vi "Dashboard Main.vi"() -> ()   [LabVIEW 2011]
uses:
  2898 Robot Code/TypeDefs/Dashboard Data TypeDef.ctl
  <vilib>/Rock Robotics/WPI/Camera/WPI_CameraImageSize.ctl
panel:
  out "Mode":enum8{"Tele-Op", "Auto", ""}(ring)=enum."Auto"
  in  "Hybrid Close":T1={"Left"=138, "Top"=0, "Right"=209, "Bottom"=45}
  out "Kinect Angle":dbl
  out "FIRE!!!!!":bool
  out "Arms in Correct Position?":bool
  out "Right Y":dbl(slide) scale=-1.0..1.0
  out "Distance Away from Player (Feet)":dbl
  out "Left Y":dbl(slide) scale=-1.0..1.0
  out "Is Kinect Override Enabled?":bool
  out "Is Kinect Enabled?":bool
  in  "Teleop":T1={"Left"=144, "Top"=36, "Right"=201, "Bottom"=76}
  in  "stop":bool
  out "Aligning Mode?":bool
  out "Bridge Mode?":bool
  in  "Ball Count Down":bool
  in  "Ball Count Up":bool
  out "Number of Balls":i32=2
  out "Shooting Manual Override?":bool
  in  "Autonomous Delay":dbl
  in  "Autonomcous Mode":T2(ring) caption="Autonomous Mode"
  out "Ball Collection":bool
  out "Shooter":bool=TRUE
  out "Shooter At Speed?":bool
  out "Ball Camera":T3(plugin-control)
  out "Image Error Message 2":string="Timeout in Camera Communications"
  out "Target Camera":T3(plugin-control)
  out "Dashboard Datatype Warning":string="Warning: The Dashboard Datatype used by the robot project and this dashboard do not match.\nSee diagram for more details."
  out "Robot IP Address":string="10.15.10.2"
  out "Image Error Message":string="Timeout in Camera Communications"
  # "Communications"
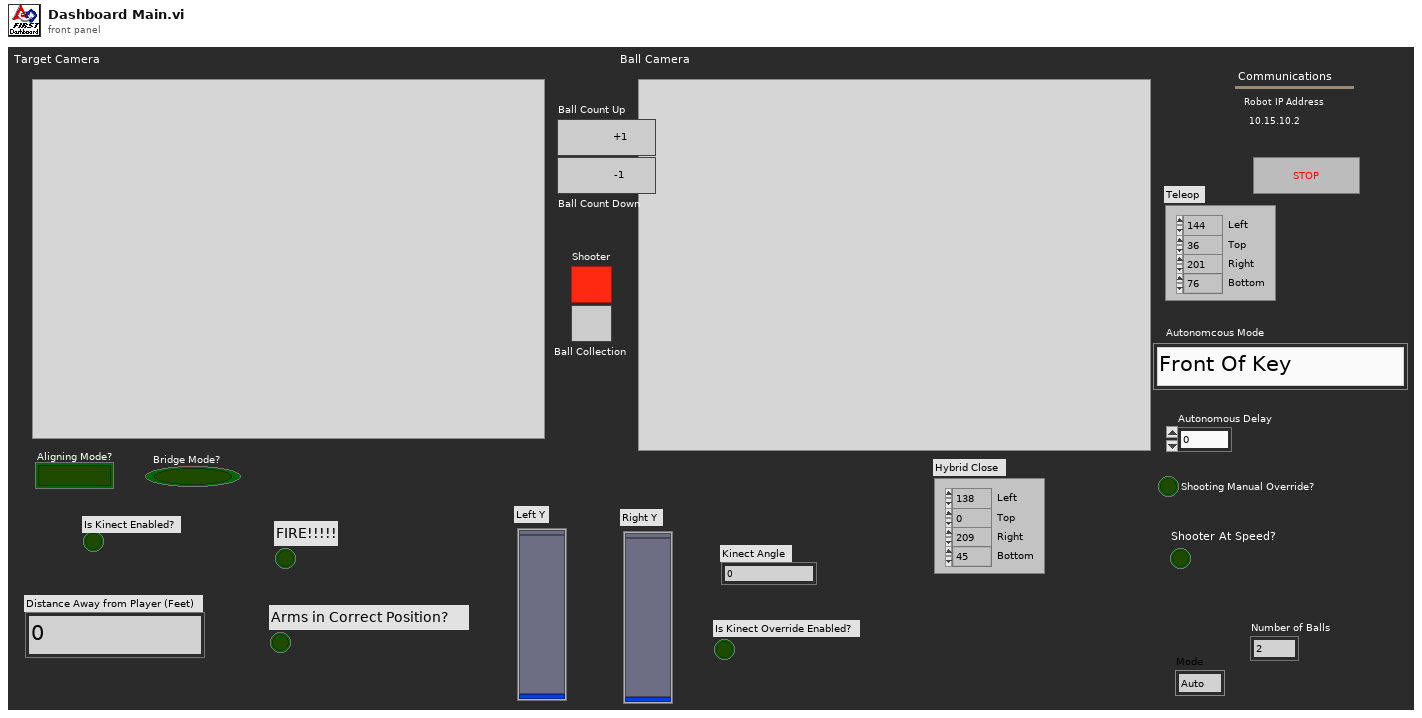
[diagram p1: front panel]
types:
  T1 = cluster{"Left":i32, "Top":i32, "Right":i32, "Bottom":i32}
  T2 = enum16{"Front Of Key", "Middle of Key (SEA)", "Back of Key", "Bridge", "Disable"}
  T3 = typedef "IMAQ Image.ctl" = refnum<image>
  T4 = typedef "Image Type" = u32
  T5 = cluster{"Ball Count Up":bool, "Ball Count Down":bool}
  T6 = cluster{"Autonomous Delay":dbl, "Autonomcous Mode":enum16{"Front Of Key", "Middle of Key (SEA)", "Back of Key", "Bridge", "Disable"}}
  T7 = cluster{cluster{"Ball Count Up":bool, "Ball Count Down":bool}, cluster{"Autonomous Delay":dbl, "Autonomcous Mode":enum16{"Front Of Key", "Middle of Key (SEA)", "Back of Key", "Bridge", "Disable"}}}
  T8 = typedef "Vector4.ctl" = cluster{"x":sgl, "y":sgl, "z":sgl, "w":sgl}
  T9 = typedef "SkeletonTrackState.ctl" = enum32{"NotTracked", "PositionOnly", "Tracked"}
  T10 = typedef "WPI_JoystickDeviceDataRaw.ctl" = cluster{"axis 1":i8, "axis 2":i8, "axis 3":i8, "axis 4":i8, "axis 5":i8, "axis 6":i8, "Buttons":u16}
  T11 = cluster{cluster{"Version String":string, "Number of Players":i8, "Flags":u32, "FloorClipPlane":T8, "Gravity Normal":cluster{"x":sgl, "y":sgl, "z":sgl}}, cluster{"TrackingState":u8[], "Overall Position":cluster{"x":sgl, "y":sgl, "z":sgl}, "Quality":u32, "TrackState":T9}, "Skeleton Vertices":cluster{"x":sgl, "y":sgl, "z":sgl}[], "Joystick":T10, "Joystick 2":T10, "Custom Data":string}
  T12 = typedef "Dashboard Data TypeDef.ctl" = cluster{"Number of Balls":i32, "Shooting Manual Override?":bool, "Bridge Mode?":bool, "Shooter":bool, "Shooter At Speed?":bool, "Aligning Mode?":bool}
  T13 = cluster{"Competition mode":bool, "Robot Link":bool, "Autonomous":bool, "Enabled":bool, "E-Stop":bool}
  T14 = typedef "WPI_CameraImageSize.ctl" = enum16{"640x480", "320x240", "160x120"}
  T15 = cluster{"fps":i32, "compression":i32, "Image Size":T14}
  T16 = typedef "LVRectTypeDef.ctl" = cluster{"left":i16, "top":i16, "right":i16, "bottom":i16}
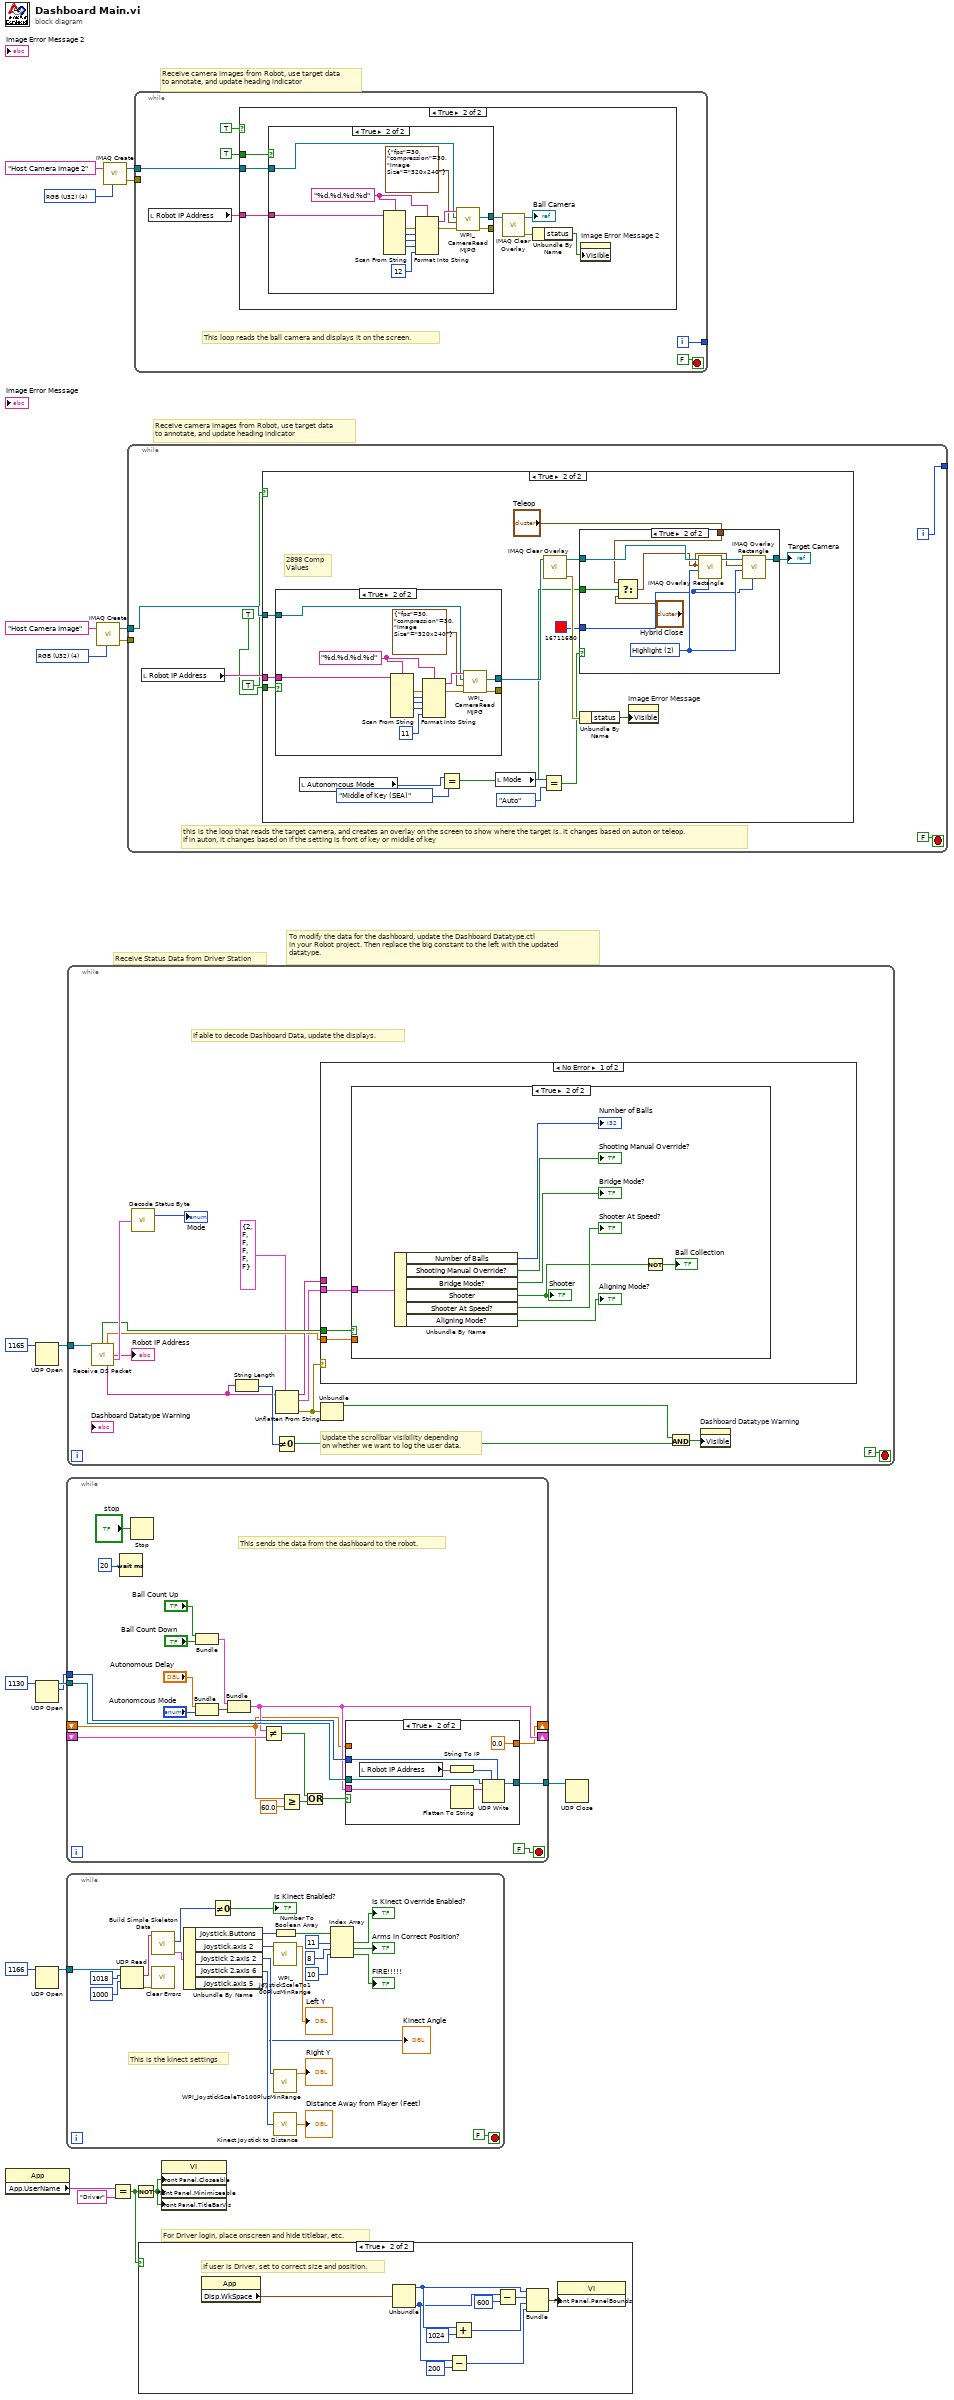
[diagram p0: block diagram]
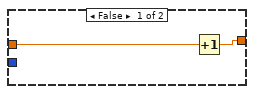
[diagram p2: hidden frame]
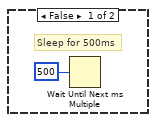
[diagram p3: hidden frame]
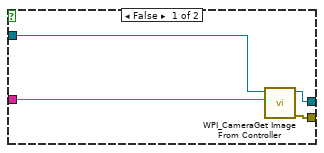
[diagram p4: hidden frame]
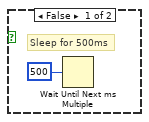
[diagram p8: hidden frame]
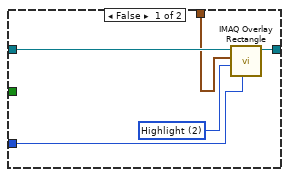
[diagram p9: hidden frame]
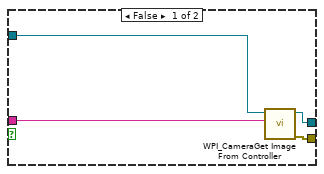
[diagram p10: hidden frame]
diagram:
  w8 = T4 4 items=["Grayscale (U8)", "Grayscale (I16)", "Grayscale (SGL)", "Complex (CSG)", "RGB (U32)", "HSL (U32)", "RGB (U64)"] ("Image Type")
  w18 = T4 4 items=["Grayscale (U8)", "Grayscale (I16)", "Grayscale (SGL)", "Complex (CSG)", "RGB (U32)", "HSL (U32)", "RGB (U64)"] ("Image Type")
  # "Receive camera images from Robot, use target data\nto annotate, and update heading indicator"
  # "For Driver login, place onscreen and hide titlebar, etc."
  # "To modify the data for the dashboard, update the Dashboard Datatype.ctl\nin your Robot project. Then replace the big constant to the left with the updated\ndatatype."
  # "Receive Status Data from Driver Station"
  # "Receive camera images from Robot, use target data\nto annotate, and update heading indicator"
  n1 = property class="App"() -> ("App.UserName"=w13:string)  [unwired: 2 in, 2 out]
  n2 = UDP Open(11:u16 1165 ("port")) -> (port=w19:refnum<k16>)  [unwired: 2 in, 4 out]
  n3 = UDP Open(11:u16 1130 ("port")) -> (port=w7:refnum<k16>, 2:w6:u16)  [unwired: 4 in, 1 out]
  n4 = UDP Open(11:u16 1166 ("port")) -> (port=w1:refnum<k16>)  [unwired: 2 in, 4 out]
  n5 = while {
    tunnel: w7 -> [w36]
    tunnel: w6 -> [w35]
    tunnel: [w34] -> w5
    shift-right: [w33] -> _
    shift-left: _ -> [w32]
    shift-right: [w29] -> _
    shift-left: _ -> [w26]
    stop <- FALSE stop-if-true
    # "This sends the data from the dashboard to the robot."
    n6 = Wait (ms)(milliseconds to wait=u32 20) -> ()  [unwired: 1 out]
    n7 = Stop(stop? (T)="stop") -> ()
    n8 = Bundle("Ball Count Up"="Ball Count Up", "Ball Count Down"="Ball Count Down") -> (w38:T5)  [unwired: 1 in]
    n9 = Bundle("Autonomous Delay"="Autonomous Delay", "Autonomcous Mode"="Autonomcous Mode") -> (w37:T6)  [unwired: 1 in]
    n10 = Bundle(w38, w37) -> (w33:T7)  [unwired: 1 in]
    n11 = Not Equal?(x=w33, y=w32) -> (x != y?=w25:bool)
    n12 = Greater Or Equal?(x=w26, y=60.0) -> (x >= y?=w27:bool)
    n13 = Or(x=w25, y=w27) -> (x .or. y?=w24:bool)
    n14 = case shown="True" w24 {
      tunnel: w33 -> [_ w50]
      tunnel: w36 -> [_ w48]
      tunnel: w35 -> [_ w47]
      tunnel: [_ w46] -> w34
      tunnel: [w42 0.0] -> w29
      tunnel: w26 -> [w41 _]
      frame False {
        n15 = Increment(x=w41) -> (x+1=w42:dbl)
      }
      frame True {
        n16 = local read "Robot IP Address"() -> (w44:string)
        n17 = String To IP(1:w44) -> (0:w45:u32)
        n18 = Flatten To String(anything=w50) -> (data string=w49:string)  [unwired: 3 in, 2 out]
        n19 = UDP Write(address=w45, port or service name=w47, connection ID=w48, data in=w49) -> (3:w46:refnum<k16>)  [unwired: 2 in, 1 out]
      }
    }
  }
  n20 = while {
    tunnel: w1 -> [w72]
    stop <- FALSE stop-if-true
    # "This is the kinect settings"
    n21 = UDP Read(connection ID=w72, max size (548)=1018 ("bytes to read"), timeout ms (25000)=1000) -> (data out=w71:string, error out=w62:errorcluster)  [unwired: 1 in, 3 out]
    n22 = call "Build Simple Skeleton Data.vi"("data out"=w71) -> ("Kinect Outputs"=w68:T11, "NumPlayers"=w70:i8)  [unwired: 6 in, 3 out]
    n23 = call <vilib>:"Clear Errors.vi"("error in (no error)"=w62) -> ()  [unwired: 6 in, 1 out]
    n24 = Unbundle By Name(w68) -> ("Joystick.Buttons"=w67:u16, "Joystick.axis 2"=w59:i8, "Joystick 2.axis 2"=w58:i8, "Joystick 2.axis 6"=w61:i8, "Joystick.axis 5"=→"Kinect Angle":i8)
    n25 = Not Equal To 0?(x=w70) -> (x != 0?=→"Is Kinect Enabled?":bool)
    n26 = call <vilib>:"WPI_JoystickScaleTo100PlusMinRange.vi"("RawValue"=w59) -> ("ScaledToPercentRange"=→"Left Y":dbl)  [unwired: 1 in, 9 out]
    n27 = call <vilib>:"WPI_JoystickScaleTo100PlusMinRange.vi"("RawValue"=w58) -> ("ScaledToPercentRange"=→"Right Y":dbl)  [unwired: 1 in, 9 out]
    n28 = call "Kinect Joystick to Distance.vi"("Input"=w61) -> ("Output"=→"Distance Away from Player (Feet)":dbl)
    n29 = Number To Boolean Array(number=w67) -> (Boolean array=w66:bool[])
    n30 = Index Array(array=w66, index #1=11 ("index"), index #2=8 ("index"), index #3=10 ("index")) -> (element #1=→"Is Kinect Override Enabled?":bool, element #2=→"Arms in Correct Position?":bool, element #3=→"FIRE!!!!!":bool)
  }
  n31 = while {
    tunnel: w19 -> [w89]
    stop <- FALSE stop-if-true
    # "Update the scrollbar visibility depending\non whether we want to log the user data."
    # "If able to decode Dashboard Data, update the displays."
    n32 = call "Receive DS Packet.vi"("Recv Socket"=w89) -> ("New Dashboard Data"=w87:bool, "Battery"=w80:sgl, "Robot IP Address"=→"Robot IP Address":string, "Status"=w90:T13, "High Priority User Data"=w77:string)  [unwired: 1 in, 9 out]
    n33 = call "Decode Status Byte.vi"("Status Byte"=w90) -> ("Mode"=→"Mode":enum8{"Tele-Op", "Auto", ""})  [unwired: 1 out]
    n34 = String Length(string=w77) -> (length=w82:i32)
    n35 = Not Equal To 0?(x=w82) -> (x != 0?=w85:bool)
    n36 = Unflatten From String(type=T12 {"Number of Balls"=2, "Shooting Manual Override?"=FALSE, "Bridge Mode?"=FALSE, "Shooter"=FALSE, "Shooter At Speed?"=FALSE, "Aligning Mode?"=FALSE} ("Cluster"), binary string=w77) -> (rest of the binary string=w83:string, value=w79:T12, error out=w88:errorcluster)  [unwired: 1 in, 2 out]
    n37 = case shown="No Error" w88 {
      tunnel: w87 -> [w93 _]
      tunnel: w83 -> [_ _]
      tunnel: w80 -> [w92 _]
      tunnel: w79 -> [w91 _]
      frame No Error {
        n38 = case shown="True" w93 {
          tunnel: w92 -> [_ _]
          tunnel: w91 -> [_ w101]
          frame False {
            # "Don't update if the robot hasn't sent new data"
          }
          frame True {
            n39 = Unbundle By Name(w101) -> ("Number of Balls"=→"Number of Balls":i32, "Shooting Manual Override?"=→"Shooting Manual Override?":bool, "Bridge Mode?"=→"Bridge Mode?":bool, "Shooter"=w95:bool, "Shooter At Speed?"=→"Shooter At Speed?":bool, "Aligning Mode?"=→"Aligning Mode?":bool)
            "Shooter" <- w95
            n40 = Not(x=w95) -> (.not. x?=→"Ball Collection":bool)
          }
        }
      }
      frame Error {
        # "Your datatypes don't match. The Dashboard Datatype.ctl in your Robot project\nand the big constant to the left of the loop need to match."
      }
    }
    n41 = Unbundle(w88) -> ("status"=w84:bool)  [unwired: 2 out]
    n42 = And(x=w84, y=w85) -> (x .and. y?=w86:bool)
    n43 = property on="Dashboard Datatype Warning" class="Str"("Visible"=w86) -> ()  [unwired: 2 in, 2 out]
  }
  n44 = call "IMAQ Create"("Image Name"="Host Camera Image", "Image Type"=w18) -> ("New Image"=w16:T3, "error out"=w15:errorcluster)  [unwired: 2 in, 1 out]
  n45 = call "IMAQ Create"("Image Name"="Host Camera Image 2", "Image Type"=w8) -> ("New Image"=w10:T3, "error out"=w11:errorcluster)  [unwired: 2 in, 1 out]
  n46 = Equal?(x=w13, y="Driver") -> (x = y?=w12:bool)
  n47 = while {
    tunnel: w16 -> [w105]
    tunnel: w15 -> [_]
    tunnel: [w103] -> _
    i -> [w103]
    stop <- FALSE stop-if-true
    # "this is the loop that reads the target camera, and creates an overlay on the screen to show where the target is. It changes based on auton or teleop.\nIf in auton, it changes based on if the setting is front of key or middle of key"
    n48 = local read "Robot IP Address"() -> (w106:string)
    n49 = case shown="True" TRUE {
      tunnel: w106 -> [_ w124]
      tunnel: w105 -> [_ w123]
      tunnel: TRUE -> [_ w119]
      frame False {
        # "Sleep for 500ms"
        n50 = Wait Until Next ms Multiple(millisecond multiple=u32 500) -> ()  [unwired: 1 out]
      }
      frame True {
        # "2898 Comp\nValues"
        n51 = case shown="True" w119 {
          tunnel: w123 -> [w141 w149]
          tunnel: [w139 w147] -> _
          tunnel: [w140 w148] -> w120
          tunnel: w124 -> [w142 w152]
          frame False {
            n52 = call <vilib>:"WPI_CameraGet Image From Controller.vi"("Controller Address"=w142, "Image"=w141) -> ("error out"=w139:errorcluster, "Image Out"=w140:T3)  [unwired: 2 in, 6 out]
          }
          frame True {
            w144 = "%d.%d.%d.%d" ("format string")
            n53 = Scan From String(format string=w144, input string=w152) -> (error out=w151:errorcluster, output 1=w153:i32, output 2=w154:i32, output 3=w155:i32)  [unwired: 2 in, 7 out]
            n54 = Format Into String(format string=w144, error in=w151, w153, w154, w155, 11 ("IP Suffix:")) -> (resulting string=w150:string, error out=w146:errorcluster)  [unwired: 1 in]
            n55 = call <vilib>:"WPI_CameraRead MJPG.vi"("error in"=w146, "Camera Settings"=T15 {"fps"=30, "compression"=30, "Image Size"=enum."320x240"}, "Image"=w149, "address"=w150) -> ("error out"=w147:errorcluster, "Image Out"=w148:T3)  [unwired: 6 in]
          }
        }
        n56 = local read "Autonomcous Mode"() -> (w111:T2)
        n57 = Equal?(x=w111, y=T2."Middle of Key (SEA)") -> (x = y?=w109:bool)
        n58 = local read "Mode"() -> (w118:enum8{"Tele-Op", "Auto", ""})
        n59 = Equal?(x=w118, y=enum8{"Tele-Op", "Auto", ""}."Auto") -> (x = y?=w116:bool)
        n60 = call "IMAQ Clear Overlay"("Image"=w120) -> ("error out"=w121:errorcluster, "Image Out"=w115:T3)  [unwired: 2 in, 7 out]
        n61 = case shown="True" w116 {
          tunnel: [w127 w136] -> w114
          tunnel: w115 -> [w128 w134]
          tunnel: u32 16711680 ("Color") -> [w126 w135]
          tunnel: "Teleop" -> [w125 w131]
          tunnel: w109 -> [_ w130]
          frame False {
            w129 = u32 2 items=["Frame", "Fill", "Highlight"] ("Drawing Mode (Frame)")
            n62 = call "IMAQ Overlay Rectangle"("Color"=w126, "Drawing Mode (Frame)"=w129, "Rectangle"=w125, "Image"=w128) -> ("Image Out"=w127:T3)  [unwired: 6 in, 1 out]
          }
          frame True {
            w137 = u32 2 items=["Frame", "Fill", "Highlight"] ("Drawing Mode (Frame)")
            n63 = Select(t=w131, s=w130, f="Hybrid Close") -> (s? t:f=w133:T1)
            n64 = call "IMAQ Overlay Rectangle"("Color"=w135, "Drawing Mode (Frame)"=w137, "Rectangle"=w133, "Image"=w134) -> ("Image Out"=w138:T3)  [unwired: 6 in, 1 out]
            n65 = call "IMAQ Overlay Rectangle"("Color"=w135, "Drawing Mode (Frame)"=w137, "Rectangle"=w133, "Image"=w138) -> ("Image Out"=w136:T3)  [unwired: 6 in, 1 out]
          }
        }
        "Target Camera" <- w114
        n66 = Unbundle By Name(w121) -> ("status"=w122:bool)
        n67 = property on="Image Error Message" class="Str"("Visible"=w122) -> ()  [unwired: 2 in, 2 out]
      }
    }
  }
  n68 = while {
    tunnel: w10 -> [w159]
    tunnel: w11 -> [_]
    tunnel: [w157] -> _
    i -> [w157]
    stop <- FALSE stop-if-true
    # "This loop reads the ball camera and displays it on the screen."
    n69 = local read "Robot IP Address"() -> (w160:string)
    n70 = case shown="True" TRUE {
      tunnel: w160 -> [_ w169]
      tunnel: w159 -> [_ w168]
      tunnel: TRUE -> [_ w163]
      frame False {
        # "Sleep for 500ms"
        n71 = Wait Until Next ms Multiple(millisecond multiple=u32 500) -> ()  [unwired: 1 out]
      }
      frame True {
        n72 = case shown="True" w163 {
          tunnel: w168 -> [w172 w180]
          tunnel: [w170 w178] -> _
          tunnel: [w171 w179] -> w165
          tunnel: w169 -> [w173 w183]
          frame False {
            n73 = call <vilib>:"WPI_CameraGet Image From Controller.vi"("Controller Address"=w173, "Image"=w172) -> ("error out"=w170:errorcluster, "Image Out"=w171:T3)  [unwired: 2 in, 6 out]
          }
          frame True {
            w175 = "%d.%d.%d.%d" ("format string")
            n74 = Scan From String(format string=w175, input string=w183) -> (error out=w182:errorcluster, output 1=w184:i32, output 2=w185:i32, output 3=w186:i32)  [unwired: 2 in, 7 out]
            n75 = Format Into String(format string=w175, error in=w182, w184, w185, w186, 12 ("IP Suffix:")) -> (resulting string=w181:string, error out=w177:errorcluster)  [unwired: 1 in]
            n76 = call <vilib>:"WPI_CameraRead MJPG.vi"("error in"=w177, "Camera Settings"=T15 {"fps"=30, "compression"=30, "Image Size"=enum."320x240"}, "Image"=w180, "address"=w181) -> ("error out"=w178:errorcluster, "Image Out"=w179:T3)  [unwired: 6 in]
          }
        }
        n77 = call "IMAQ Clear Overlay"("Image"=w165) -> ("error out"=w166:errorcluster, "Image Out"=→"Ball Camera":T3)  [unwired: 2 in, 7 out]
        n78 = Unbundle By Name(w166) -> ("status"=w167:bool)
        n79 = property on="Image Error Message 2" class="Str"("Visible"=w167) -> ()  [unwired: 2 in, 2 out]
      }
    }
  }
  n80 = Not(x=w12) -> (.not. x?=w3:bool)
  n81 = case shown="True" w12 {
    frame False {
    }
    frame True {
      # "If user is Driver, set to correct size and position."
      n82 = property class="App"() -> ("Disp.WkSpace"=w196:T16)  [unwired: 2 in, 2 out]
      n83 = Unbundle(w196) -> ("left"=w191:i16, "bottom"=w187:i16)  [unwired: 2 out]
      n84 = Subtract(x=w187, y=200) -> (x-y=w188:i32)
      n85 = Add(x=w191, y=1024) -> (x+y=w192:i32)
      n86 = Subtract(x=w187, y=600) -> (x-y=w193:i32)
      n87 = Bundle("left"=w191, w193, w192, w188) -> (w195:cluster{"left":i16, i32, i32, i32})  [unwired: 1 out]
      n88 = property class="VI"("Front Panel.PanelBounds"=w195) -> ()  [unwired: 2 in, 2 out]
    }
  }
  n89 = property class="VI"("Front Panel.Closeable"=w3, "Front Panel.Minimizeable"=w3, "Front Panel.TitleBarVis"=w3) -> ()  [unwired: 2 in, 2 out]
  n90 = UDP Close(connection ID=w5) -> ()  [unwired: 1 in, 2 out]
